vi "Encoders_pickup.vi"(4 "Reset Encoder?":bool, 5 "B Channel":T1=enum."DIO 2", 6 "A Channel":T1, 7 "State Control":enum16{"Open", "Run", "End"}(ring)) -> (0 "Encoder Alarm Status":string, 1 "Encoder Rate (distance/sec)":dbl, 2 "Encoder Direction":string, 3 "Encoder Degrees":dbl)   [LabVIEW 2013]
uses:
  <vilib>/Rock Robotics/WPI/Encoder/WPI_EncoderType.ctl
  <vilib>/Rock Robotics/SystemInterfaces/DIO/FPGA_DIOChannel.ctl
  <vilib>/Rock Robotics/WPI/Counter/WPI_CounterDigitalInputToDigitalSource.vi
panel:
  in  "Number Samples to Average":u8=1 min=1 max=128
  in  "Invert Direction":bool
  in  "Decoding Type":T2=enum."4x"
  in  "DistancePerCount":dbl=1.0
  in  "Minimum Rate":dbl=20.0
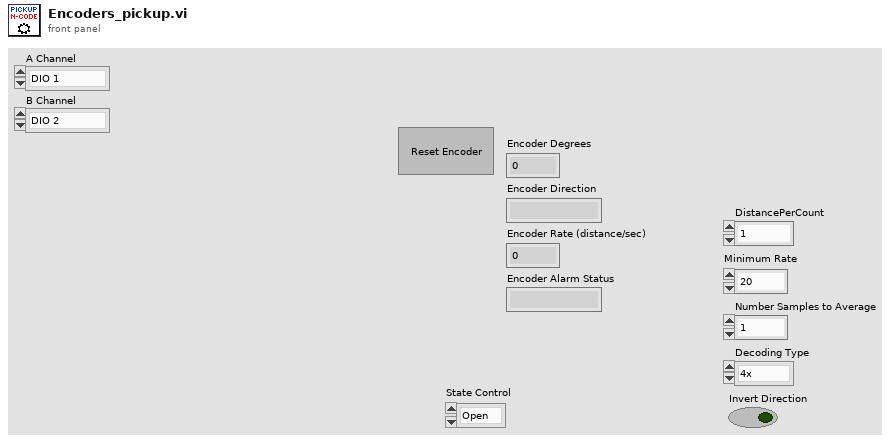
[diagram p1: front panel]
types:
  T1 = typedef "FPGA_DIOChannel.ctl" = enum8{"DIO 1", "DIO 2", "DIO 3", "DIO 4", "DIO 5", "DIO 6", "DIO 7", "DIO 8", "DIO 9", "DIO 10", "DIO 11", "DIO 12", "DIO 13", "DIO 14", "Invalid"}
  T2 = typedef "WPI_EncoderType.ctl" = enum16{"1x", "2x", "4x"}
  T3 = typedef "WPI_DigitalInputDevRef.ctl" = cluster{"DevStatus":errorcluster, "DIO Channel":T1, "Digital Module":T4}
  T4 = typedef "FPGA_TypedefDigitalModule.ctl" = enum16{"Digital Module 1", "Digital Module 2"}
  T5 = typedef "FPGA_CounterEncoderSourceConvertionLVSourceType.ctl" = cluster{"DevStatus":errorcluster, "AnalogTriggerMode?":bool, "DigitalMode":cluster{"Digital Module":T4, "DIO Channel":T6}, "AnalogTriggerMode":cluster{"AnalogTriggerIndex":T7, "OutputType":T8}}
  T6 = typedef "FPGA_DIODigitalSourceChannel.ctl" = enum8{"DIO 1", "DIO 2", "DIO 3", "DIO 4", "DIO 5", "DIO 6", "DIO 7", "DIO 8", "DIO 9", "DIO 10", "DIO 11", "DIO 12", "DIO 13", "DIO 14", "Disabled"}
  T7 = typedef "FPGA_AnalogTriggerIndex.ctl" = enum8{"Trig 0", "Trig 1", "Trig 2", "Trig 3", "Trig 4", "Trig 5", "Trig 6", "Trig 7", "Invalid"}
  T8 = typedef "FPGA_AnalogTriggerOutType.ctl" = enum16{"InWindow", "TriggerState", "Rising", "Falling"}
  T9 = typedef "WPI_EncoderDevRef.ctl" = cluster{"DevStatus":errorcluster, "EncoderIndex":T10, "CounterIndex":T11, "DistancePerCount":dbl, "Decoding Type":T2}
  T10 = typedef "FPGA_EncoderIdx.ctl" = enum8{"Enc 0", "Enc 1", "Enc 2", "Enc 3", "Invalid"}
  T11 = typedef "FPGA_CounterCtrSystemIndex.ctl" = enum8{"Ctr 0", "Ctr 1", "Ctr 2", "Ctr 3", "Ctr 4", "Ctr 5", "Ctr 6", "Ctr 7", "Invalid"}
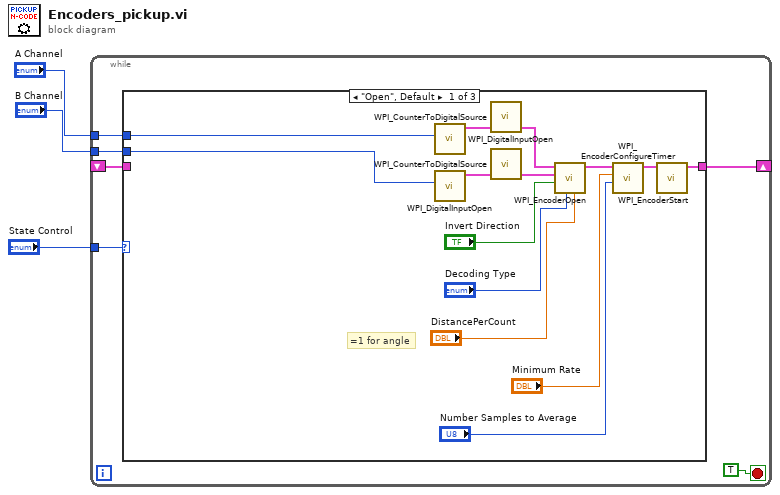
[diagram p0: block diagram]
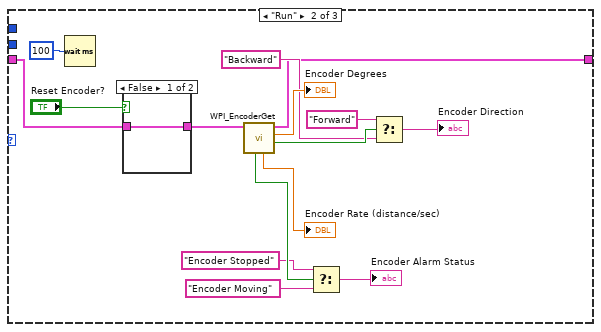
[diagram p2: hidden frame]
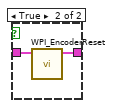
[diagram p3: hidden frame]
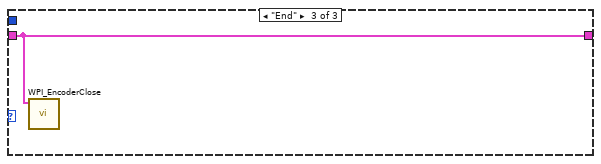
[diagram p4: hidden frame]
diagram:
  n1 = while {
    tunnel: "State Control" -> [w9]
    shift-right: [w7] -> _
    shift-left: _ -> [w6]
    tunnel: "A Channel" -> [w5]
    tunnel: "B Channel" -> [w4]
    stop <- TRUE stop-if-true
    n2 = case shown="\"Open\", Default" w9 {
      tunnel: [w12 w26 w42] -> w7
      tunnel: w6 -> [_ w25 w42]
      tunnel: w5 -> [w11 _ _]
      tunnel: w4 -> [w10 _ _]
      frame "Open", Default {
        # "=1 for angle"
        n3 = call <vilib>:"WPI_DigitalInputOpen.vi"("DIO Channel"=w11) -> ("DigitalInputDevRef"=w21:T3)  [unwired: 2 in, 8 out]
        n4 = call <vilib>:"WPI_DigitalInputOpen.vi"("DIO Channel"=w10) -> ("DigitalInputDevRef"=w22:T3)  [unwired: 2 in, 8 out]
        n5 = call-poly <vilib>:"WPI_CounterToDigitalSource.vi"("DigitalInputDevRef"=w21) -> ("Digital Source"=w20:T5)  [unwired: 6 out]
        n6 = call-poly <vilib>:"WPI_CounterToDigitalSource.vi"("DigitalInputDevRef"=w22) -> ("Digital Source"=w23:T5)  [unwired: 6 out]
        n7 = call <vilib>:"WPI_EncoderOpen.vi"("DistancePerCount"="DistancePerCount", "Decoding Type"="Decoding Type", "Invert Direction (False)"="Invert Direction", "BSource"=w23, "ASource"=w20) -> ("EncoderDevRef"=w15:T9)  [unwired: 3 in, 3 out]
        n8 = call <vilib>:"WPI_EncoderConfigureTimer.vi"("Number Samples to Average"="Number Samples to Average", "Minimum Rate"="Minimum Rate", "EncoderDevRef"=w15) -> ("EncoderDevRef"=w16:T9)  [unwired: 1 in, 7 out]
        n9 = call <vilib>:"WPI_EncoderStart.vi"("EncoderDevRef"=w16) -> ("EncoderDevRef"=w12:T9)  [unwired: 1 in, 9 out]
      }
      frame "Run" {
        n10 = Wait (ms)(milliseconds to wait=u32 100) -> ()  [unwired: 1 out]
        n11 = case shown="False" "Reset Encoder?" {
          tunnel: w25 -> [w39 w40]
          tunnel: [w39 w41] -> w35
          frame False {
          }
          frame True {
            n12 = call <vilib>:"WPI_EncoderReset.vi"("EncoderDevRef"=w40) -> ("EncoderDevRef"=w41:T9)  [unwired: 1 in, 9 out]
          }
        }
        n13 = call <vilib>:"WPI_EncoderGet.vi"("EncoderDevRef"=w35) -> ("Direction"=w34:bool, "Distance"=→"Encoder Degrees":dbl, "EncoderDevRef"=w26:T9, "Rate"=→"Encoder Rate (distance/sec)":dbl, "Stopped"=w33:bool)  [unwired: 1 in, 5 out]
        n14 = Select(t="Encoder Stopped", s=w33, f="Encoder Moving") -> (s? t:f=→"Encoder Alarm Status":string)
        n15 = Select(t="Forward", s=w34, f="Backward") -> (s? t:f=→"Encoder Direction":string)
      }
      frame "End" {
        n16 = call <vilib>:"WPI_EncoderClose.vi"("EncoderDevRef"=w42) -> ()  [unwired: 2 in, 9 out]
      }
    }
  }
